vi "GetRightEncoderRefnum.vi"() -> (2 "RightEncoderRefnum":string)   [LabVIEW 2016, in "DriveBase.lvclass"]
uses:
  DriveBase.lvclass
  DriveBase.lvclass/DriveBase.ctl
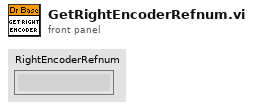
[diagram p1: front panel]
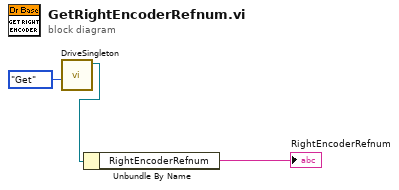
[diagram p0: block diagram]
diagram:
  n1 = call "DriveSingleton.vi"("Get/Set"=enum16{"Get", "Set"}."Get") -> ("DriveBase.lvclass 2"=w2:refnum<class "DriveBase.lvclass">)  [unwired: 9 in, 1 out]
  n2 = Unbundle By Name(w2) -> ("RightEncoderRefnum"=→"RightEncoderRefnum":string)
